vi "ReadWrite All Data.vi"(6 "Iteration":i32, 7 "Mode":T1, 8 "error in (no error)":errorcluster, 10 "ScheduledSDI":bool, 11 "RT Data in":T2 {"Label Transfer Config"."Block Data Refs"."Data Reference" format="%.0x"; "Status Config"."HWOut Dur Ref" format="%.0x"; "Status Config"."HWIn Dur Ref" format="%.0x"; "Status Config"."Error Data Ref" format="%.0x"; "HWOutput Channels"."Labels Settings"."Label" format="%.0o"; "HWInput Channels"."Labels Settings"."Label" format="%.0o"}) -> (0 "error out":errorcluster, 3 "RT Data out":T2 {"Label Transfer Config"."Block Data Refs"."Data Reference" format="%.0x"; "Status Config"."HWOut Dur Ref" format="%.0x"; "Status Config"."HWIn Dur Ref" format="%.0x"; "Status Config"."Error Data Ref" format="%.0x"; "HWOutput Channels"."Labels Settings"."Label" format="%.0o"; "HWInput Channels"."Labels Settings"."Label" format="%.0o"})   [LabVIEW 2015, in "AIT 429 Engine.lvlib"]
uses:
  AIT 429 Engine.lvlib
  RT Controls/RT Data.ctl
  RT Controls/RT HW Channel.ctl
  RT Controls/RT Label Settings.ctl
  Shared/Controls and Global/Label.ctl
  Shared/Controls and Global/transferPeriod.ctl
  RT Controls/Driver Data.ctl
  RT Controls/RT Word Settings.ctl
  <vilib>/NI Veristand/Custom Device API/Block Data Reference.ctl
  <vilib>/NI Veristand/Custom Device API/Data Reference.ctl
  RT Controls/RT Param Setting.ctl
  Shared/Controls and Global/Start Bit.ctl
  Shared/Controls and Global/Number of Bits.ctl
  Shared/Controls and Global/TransferType.ctl
  RT Controls/Error Qs.ctl
  RT Controls/Status Channels Config.ctl
  RT Controls/FIFO.ctl
  RT Controls/Label Transfer Config.ctl
  RT Controls/ReadWrite Selector.ctl
  Search Label Array for Index of Label.vi
  ReadWrite Label.vi
  Calculate Buffer Index for Label Data (AIM_AIT).vi
  Calculate Number of Labels Available to Read (AIM_AIT).vi
  Write outgoing label data.vi
  Read incoming label data.vi
  Read Parameter VS Channels.vi
  Update Parameter VS Channels.vi
  Double to selected bits.vi
  Shared/Word to double.vi
  <vilib>/NI Veristand/Custom Device API/NI VeriStand - Get Channel Values by Block Data Reference.vi
  <vilib>/NI Veristand/Custom Device API/NI VeriStand - Set Channel Values by Block Data Reference.vi
  <vilib>/NI Veristand/Custom Device API/Global Data Refs.vi
  <instrlib>/AIT 429/Public/Tx/Data/AIT 429 Set Acyclic Transfer Data.vi
  <instrlib>/AIT 429/Public/Tx/Data/AIT 429 Get Acyclic Transfer Data.vi
  <instrlib>/AIT 429/Public/Tx/Data/AIT 429 Set Block Transfer Data.vi
  <instrlib>/AIT 429/Public/Tx/Data/AIT 429 Get Block Transfer Data.vi
  <instrlib>/AIT 429/Public/Tx/Data/AIT 429 Set Scheduled Label Data.vi
  <instrlib>/AIT 429/Public/Tx/Data/AIT 429 Get Scheduled Label Data.vi
  <instrlib>/AIT 429/Public/Utility/AIT 429 Get SDI.vi
  <instrlib>/AIT 429/Public/Utility/AIT 429 Get Label.vi
  <userlib>/ARINC-429/vi/IRxChronMonChannel/Owl429_IRxChronMonChannel_read.vi
  Shared/AIT 429 Shared.lvlib
  <vilib>/NI Veristand/Custom Device API/Custom Device API.lvlib
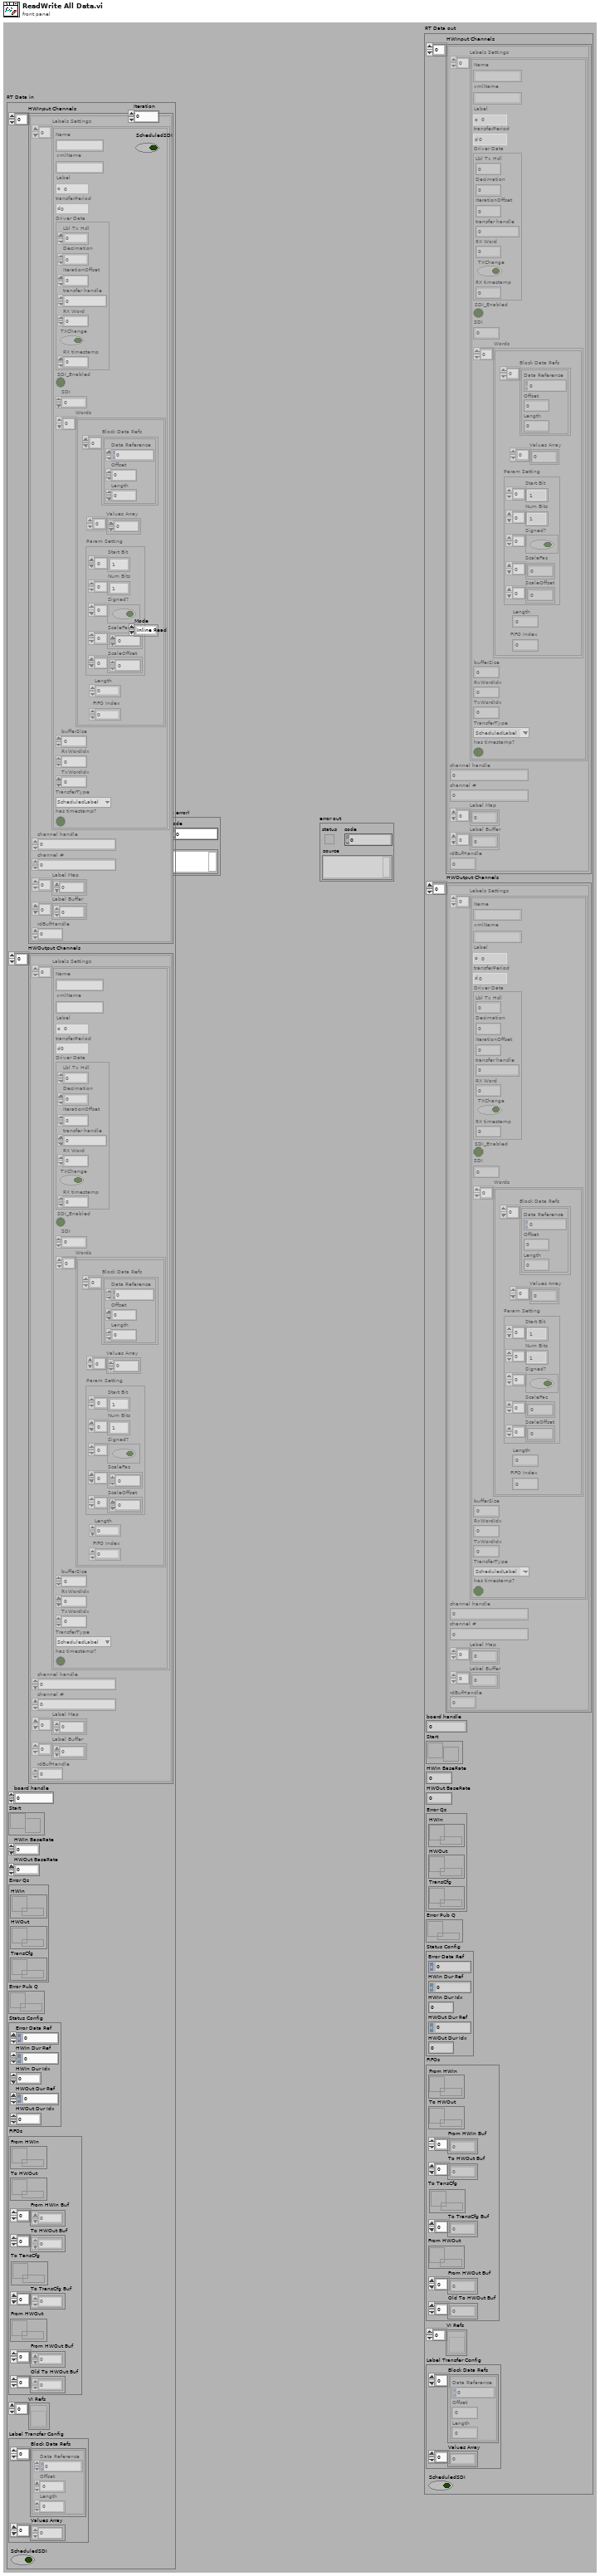
[diagram p1: front panel]
types:
  T1 = typedef "AIT 429 Engine.lvlib/ReadWrite Selector.ctl" = enum16{"Inline Read", "Inline Write", "Async HWIn", "Async HWOut"}
  T2 = typedef "AIT 429 Engine.lvlib/RT Data.ctl" = cluster{"HWInput Channels":T3[], "HWOutput Channels":T3[], "board handle":u32, "Start":refnum<notifier>, "HWIn BaseRate":i64, "HWOut BaseRate":i64, "Error Qs":T15, "Error Pub Q":refnum<queue>, "Status Config":T16, "FIFOs":T17, "VI Refs":refnum<vi>[], "Label Transfer Config":T18, "ScheduledSDI":bool}
  T3 = typedef "AIT 429 Engine.lvlib/RT HW Channel.ctl" = cluster{"Labels Settings":T4[], "channel handle":u32, "channel #":u16, "Label Map":i32[], "Label Buffer":u32[], "rdBufHandle":u32}
  T4 = typedef "AIT 429 Engine.lvlib/RT Label Settings.ctl" = cluster{"Name":string, "xmlName":string, "Label":T5, "transferPeriod":T6, "Driver Data":T7, "SDI_Enabled":bool, "SDI":u8, "Words":T8[], "bufferSize":u32, "RxWordIdx":i32, "TxWordIdx":i32, "TransferType":T14, "has timestamp?":bool}
  T5 = typedef "AIT 429 Shared.lvlib/Label.ctl" = u8
  T6 = typedef "AIT 429 Shared.lvlib/transferPeriod.ctl" = u32
  T7 = typedef "AIT 429 Engine.lvlib/Driver Data.ctl" = cluster{"Lbl Tx Hdl":u32, "Decimation":i32, "IterationOffset":i32, "transfer handle":u32, "RX Word":u32, "TXChange":bool, "RX timestamp":dbl}
  T8 = typedef "AIT 429 Engine.lvlib/RT Word Settings.ctl" = cluster{"Block Data Refs":T9[], "Values Array":dbl[], "Length":i32, "FIFO Index":i32, "Param Setting":T11}
  T9 = typedef "Custom Device API.lvlib/Block Data Reference.ctl" = cluster{"Data Reference":T10, "Offset":u64, "Length":u64}
  T10 = typedef "Custom Device API.lvlib/Data Reference.ctl" = i32
  T11 = typedef "AIT 429 Engine.lvlib/RT Param Setting.ctl" = cluster{"Start Bit":T12[], "Num Bits":T13[], "Signed?":bool[], "ScaleFac":dbl[], "ScaleOffset":dbl[]}
  T12 = typedef "AIT 429 Shared.lvlib/Start Bit.ctl" = i32
  T13 = typedef "AIT 429 Shared.lvlib/Number of Bits.ctl" = i32
  T14 = typedef "AIT 429 Shared.lvlib/TransferType.ctl" = enum16{"ScheduledLabel", "Acyclic", "Block", "Strobe"}
  T15 = typedef "AIT 429 Engine.lvlib/Error Qs.ctl" = cluster{"HWIn":refnum<queue>, "HWOut":refnum<queue>, "TransCfg":refnum<queue>}
  T16 = typedef "AIT 429 Engine.lvlib/Status Channels Config.ctl" = cluster{"Error Data Ref":T10, "HWIn Dur Ref":T10, "HWIn Dur Idx":i32, "HWOut Dur Ref":T10, "HWOut Dur Idx":i32}
  T17 = typedef "AIT 429 Engine.lvlib/FIFO.ctl" = cluster{"From HWIn":refnum<k33>, "To HWOut":refnum<k33>, "From HWIn Buf":dbl[], "To HWOut Buf":dbl[], "To TansCfg":refnum<k33>, "To TransCfg Buf":dbl[], "From HWOut":refnum<k33>, "From HWOut Buf":dbl[], "Old To HWOut Buf":dbl[]}
  T18 = typedef "AIT 429 Engine.lvlib/Label Transfer Config.ctl" = cluster{"Block Data Refs":T9[], "Values Array":dbl[]}
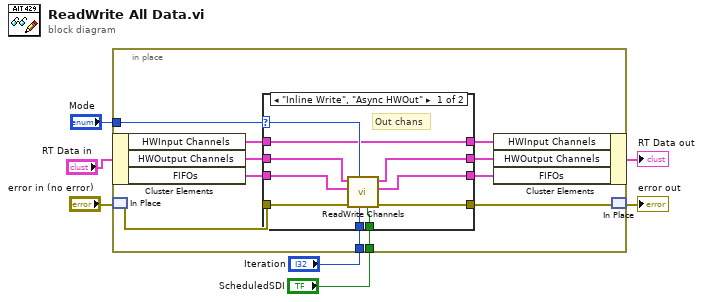
[diagram p0: block diagram]
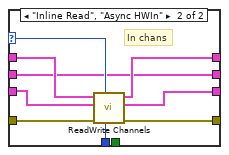
[diagram p2: hidden frame]
diagram:
  n1 = in-place {
    in-place-border: "Mode" -> [w12]
    in-place-border: "Iteration" -> [w9]
    in-place-border: "ScheduledSDI" -> [w8]
    n2 = in-place-cluster #1("RT Data in") -> ("HWInput Channels"=w18:T3[], "HWOutput Channels"=w11:T3[], "FIFOs"=w14:T17)
    n3 = in-place-match #2("error in (no error)") -> (w16:errorcluster)
    n4 = case shown="\"Inline Write\", \"Async HWOut\"" w12 {
      selector: w12 -> [w27 w33]
      tunnel: w18 -> [w23 w37]
      tunnel: [w23 w36] -> w17
      tunnel: w16 -> [w28 w35]
      tunnel: [w26 w34] -> w15
      tunnel: w14 -> [w20 w30]
      tunnel: [w21 w29] -> w13
      tunnel: w11 -> [w25 w32]
      tunnel: [w24 w32] -> w10
      tunnel: w9 -> [w22 w31]
      tunnel: w8 -> [w19 _]
      frame "Inline Write", "Async HWOut" {
        # "Out chans"
        n5 = call "ReadWrite Channels.vi"("ScheduledSDI"=w19, "Iteration"=w22, "Mode"=w27, "error in (no error)"=w28, "FIFOs In"=w20, "Channels In"=w25) -> ("error out"=w26:errorcluster, "FIFOs Out"=w21:T17, "Channels Out"=w24:T3[])  [unwired: 3 in]
      }
      frame "Inline Read", "Async HWIn" {
        # "In chans"
        n6 = call "ReadWrite Channels.vi"("Iteration"=w31, "Mode"=w33, "error in (no error)"=w35, "FIFOs In"=w30, "Channels In"=w37) -> ("error out"=w34:errorcluster, "FIFOs Out"=w29:T17, "Channels Out"=w36:T3[])  [unwired: 4 in]
      }
    }
    n7 = in-place-cluster #1("HWInput Channels"=w17, "HWOutput Channels"=w10, "FIFOs"=w13) -> (→"RT Data out":T2)
    n8 = in-place-match #2(w15) -> (→"error out":errorcluster)
  }
